vi "Create Empty Object.vi"(9 "object":refnum<class "_ISerializable.lvclass">, 10 "columns data type":string[](array[string])) -> (1 "Array 3":T1[](array[typedef]), 3 "elements by level":i32[](array[numeric]))   [LabVIEW 2018, in "Serializer.lvclass"]
uses:
  Serializer/Serializer.lvclass
  Typedefs/key-value-type cluster.ctl
  _Serializable Base Object/_ISerializable.lvclass
  demo/Implementations/Product-A.lvclass
  ORM Scripter/ORM Scripter.lvclass
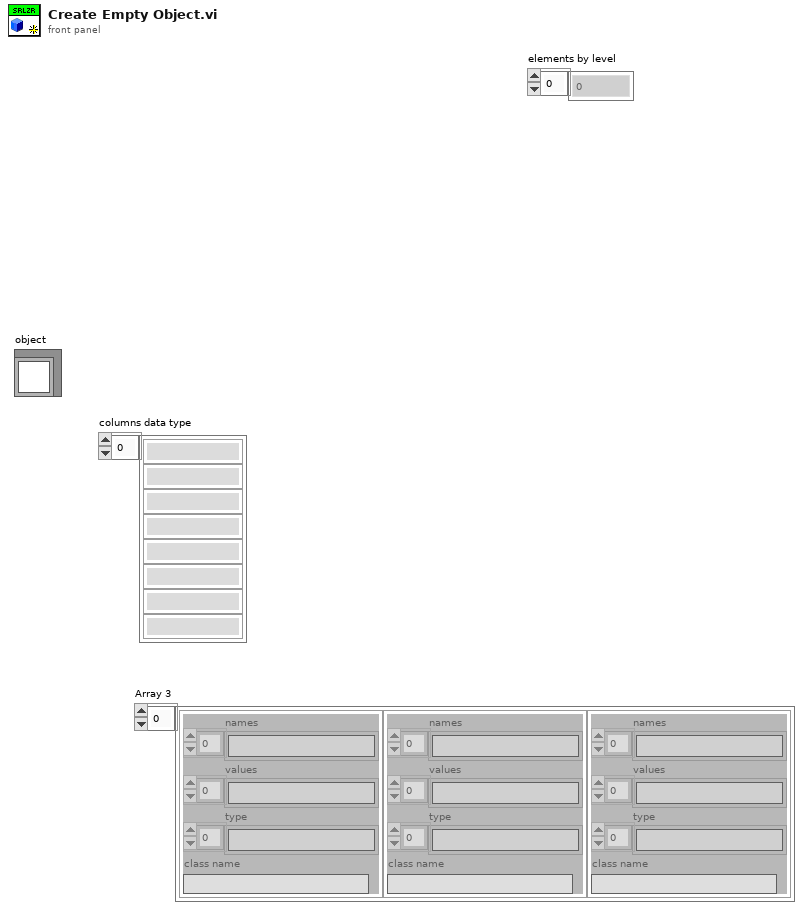
[diagram p1: front panel]
types:
  T1 = typedef "key-value-type cluster.ctl" = cluster{"names":string[], "values":string[], "type":string[], "class name":string}
  T2 = cluster{"Major":u16, "Minor":u16, "Fix":u16, "Build":u16}
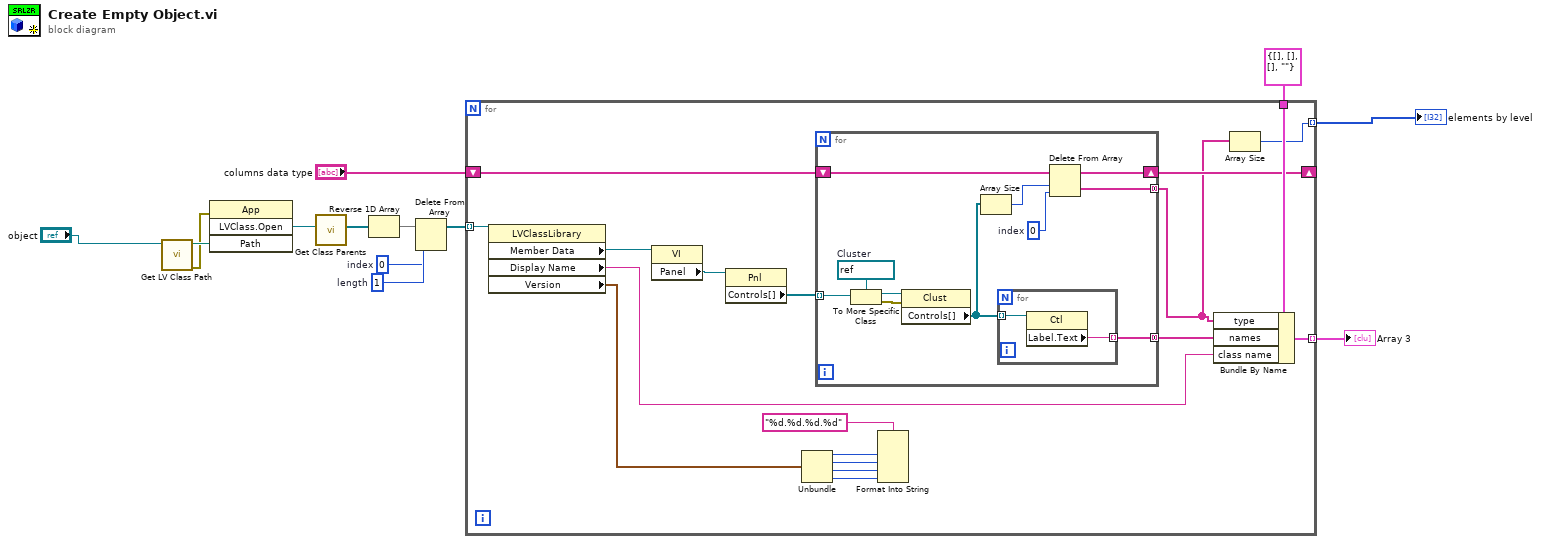
[diagram p0: block diagram]
diagram:
  w7 = 0  # index
  w8 = 1  # length
  n1 = call <vilib>:"Get LV Class Path.vi"("object"="object") -> ("error out"=w2:errorcluster, "class path"=w13:path)  [unwired: 9 in]
  n2 = invoke class="App" method="LVClass.Open"(error in=w2, "Path"=w13) -> ("LVClass.Open"=w12:refnum<vi>)  [unwired: 2 in, 3 out]
  n3 = call "Get Class Parents.vi"("LVClassLibrary in"=w12) -> ("Array"=w11:refnum<vi>[])  [unwired: 9 in, 1 out]
  n4 = Reverse 1D Array(array=w11) -> (reversed array=w10:refnum<vi>[])
  n5 = Delete From Array(array=w10, length=w8, index=w7) -> (array with subset deleted=w9:refnum<vi>[])  [unwired: 1 out]
  n6 = for {
    tunnel: w9 -> [w29] mode=indexing
    tunnel: T1 {"names"=[], "values"=[], "type"=[], "class name"=""} -> [w19]
    tunnel: [w21] -> w6 mode=indexing
    shift-right: [w17] -> _
    shift-left: "columns data type" -> [w18]
    tunnel: [w15] -> w4 mode=indexing
    n7 = property class="LVClassLibrary"(reference=w29) -> ("Member Data"=w30:refnum<vi>, "Display Name"=w22:string, "Version"=w28:T2)  [unwired: 1 in, 2 out]
    n8 = property class="VI"(reference=w30) -> ("Panel"=w31:refnum<vi>)  [unwired: 1 in, 2 out]
    n9 = property class="Pnl"(reference=w31) -> ("Controls[]"=w16:refnum<vi>[])  [unwired: 1 in, 2 out]
    n10 = Unbundle(w28) -> ("Major"=w27:u16, "Minor"=w24:u16, "Fix"=w25:u16, "Build"=w26:u16)
    n11 = for {
      tunnel: w16 -> [w38] mode=indexing
      tunnel: [w39] -> w20 mode=concatenating
      shift-right: [w33] -> w17
      shift-left: w18 -> [w37]
      tunnel: [w36] -> w14 mode=concatenating
      w32 = 0  # index
      w42 = refnum<vi> refnum  # Cluster
      n12 = To More Specific Class(target class=w42, reference=w38) -> (specific class reference=w41:refnum<vi>, error out=w40:errorcluster)  [unwired: 1 in]
      n13 = property class="Clust"(reference=w41, error in=w40) -> ("Controls[]"=w35:refnum<vi>[])  [unwired: 2 out]
      n14 = Array Size(array=w35) -> (size(s)=w34:i32)
      n15 = for {
        tunnel: w35 -> [w44] mode=indexing
        tunnel: [w43] -> w39 mode=indexing
        n16 = property class="Ctl"(reference=w44) -> ("Label.Text"=w43:string)  [unwired: 1 in, 2 out]
      }
      n17 = Delete From Array(array=w37, length=w34, index=w32) -> (deleted portion=w36:string[], array with subset deleted=w33:string[])
    }
    n18 = Format Into String(format string="%d.%d.%d.%d", w27, w24, w25, w26) -> ()  [unwired: 2 in, 2 out]
    n19 = Bundle By Name(cluster=w19, "type"=w14, "names"=w20, "class name"=w22) -> (w21:T1)
    n20 = Array Size(array=w14) -> (size(s)=w15:i32)
  }
  "Array 3" <- w6
  "elements by level" <- w4
